vi "Add Cell.vi"(8 "error in":errorcluster, 10 "Cell Address":string, 11 "Row in":refnum<k24>) -> (0 "error out":errorcluster, 2 "Cell":refnum<k24>, 3 "Row out":refnum<k24>)   [LabVIEW 2019, in "Open Xml.lvlib"]
uses:
  Open Xml.lvlib
  D:/git/Open-Xml-LabVIEW/Source/DocumentFormat.OpenXml.dll
  DocumentFormat.OpenXml.dll
  D:/git/Open-Xml-LabVIEW/Source/DocumentFormat.OpenXml.Framework.dll
  DocumentFormat.OpenXml.Framework.dll
  D:/git/Open-Xml-LabVIEW/Source/OpenXmlGenericsWrapper.dll
  OpenXmlGenericsWrapper.dll
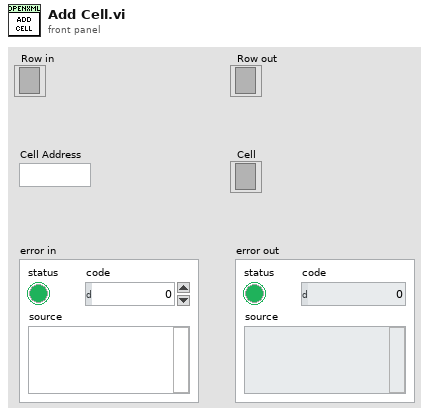
[diagram p1: front panel]
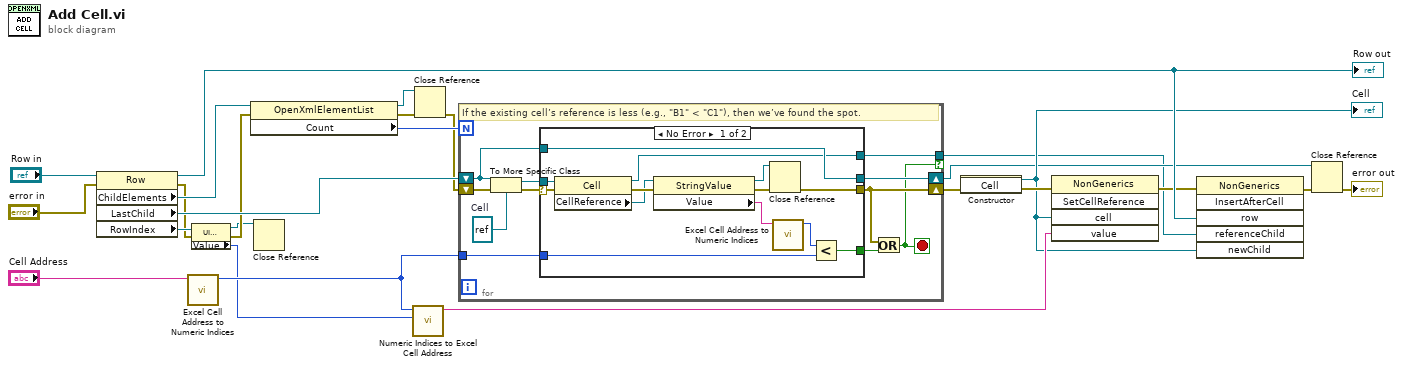
[diagram p0: block diagram]
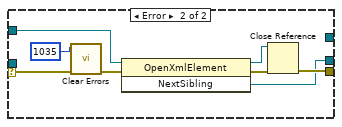
[diagram p2: hidden frame]
diagram:
  n1 = property class="Row"(reference="Row in", error in="error in") -> (reference out=w16:refnum<k24>, error out=w9:errorcluster, "ChildElements"=w24:refnum<k24>, "LastChild"=w22:refnum<k24>, "RowIndex"=w10:refnum<k24>)
  "Row out" <- w16
  n2 = call "Excel Cell Address to Numeric Indices.vi"("Cell Name"="Cell Address") -> ("Column Number"=w11:i32)  [unwired: 9 in, 1 out]
  n3 = property class="UInt32Value"(reference=w10, error in=w9) -> (reference out=w5:refnum<k24>, error out=w8:errorcluster, "Value"=w7:u32)
  n4 = property class="OpenXmlElementList"(reference=w24, error in=w8) -> (reference out=w17:refnum<k24>, error out=w21:errorcluster, "Count"=w23:i32)
  n5 = Close Reference(reference=w5) -> ()  [unwired: 1 in, 1 out]
  n6 = call "Numeric Indices to Excel Cell Address.vi"("Row"=w7, "Column"=w11) -> ("Cell Address"=w6:string)  [unwired: 9 in]
  n7 = Close Reference(reference=w17, error in (no error)=w21) -> (error out=w18:errorcluster)
  n8 = for {
    N: w23 -> [_]
    tunnel: w11 -> [w30]
    shift-right: [w29] -> w3
    shift-left: w22 -> [w31]
    tunnel: [w28] -> w2 if=w27
    shift-right: [w33] -> w13
    shift-left: w18 -> [w34]
    stop <- w27 stop-if-true
    w35 = refnum<k24> refnum  # Cell
    # "If the existing cell’s reference is less (e.g., \"B1\" < \"C1\"), then we’ve found the spot."
    n9 = To More Specific Class(target class=w35, reference=w31, error in=w34) -> (specific class reference=w32:refnum<k24>, error out=w36:errorcluster)
    n10 = case shown="No Error" w36 {
      selector: w36 -> [w49 w57]
      tunnel: [w38 w51] -> w33
      tunnel: w32 -> [w48 _]
      tunnel: w31 -> [w40 w54]
      tunnel: w30 -> [w44 _]
      tunnel: [w41 _] -> w26
      tunnel: [w40 w50] -> w29
      tunnel: [w39 _] -> w28
      frame No Error {
        n11 = property class="Cell"(reference=w48, error in=w49) -> (reference out=w39:refnum<k24>, error out=w47:errorcluster, "CellReference"=w46:refnum<k24>)
        n12 = property class="StringValue"(reference=w46, error in=w47) -> (reference out=w37:refnum<k24>, error out=w43:errorcluster, "Value"=w45:string)
        n13 = Close Reference(reference=w37, error in (no error)=w43) -> (error out=w38:errorcluster)
        n14 = call "Excel Cell Address to Numeric Indices.vi"("Cell Name"=w45) -> ("Column Number"=w42:i32)  [unwired: 9 in, 1 out]
        n15 = Less?(x=w42, y=w44) -> (x < y?=w41:bool)
      }
      frame Error {
        n16 = call <vilib>:"Clear Errors.vi"("error in (no error)"=w57, "specific error code to clear (0: all)"=1035) -> ("error out"=w55:errorcluster)  [unwired: 4 in, 1 out]
        n17 = invoke class="OpenXmlElement" method="NextSibling"(reference=w54, error in=w55) -> (reference out=w53:refnum<k24>, error out=w52:errorcluster, "NextSibling"=w50:refnum<k24>)  [unwired: 1 in]
        n18 = Close Reference(reference=w53, error in (no error)=w52) -> (error out=w51:errorcluster)
      }
    }
    n19 = Or(x=w33, y=w26) -> (x .or. y?=w27:bool)
  }
  n20 = constructor class="Cell"(error in=w13) -> (reference out=w4:refnum<k24>, error out=w20:errorcluster)  [unwired: 2 in, 1 out]
  "Cell" <- w4
  n21 = invoke class="NonGenerics" method="SetCellReference"(error in=w20, "cell"=w4, "value"=w6) -> (error out=w12:errorcluster)  [unwired: 2 in, 4 out]
  n22 = invoke class="NonGenerics" method="InsertAfterCell"(error in=w12, "row"=w16, "referenceChild"=w2, "newChild"=w4) -> (error out=w14:errorcluster)  [unwired: 2 in, 5 out]
  n23 = Close Reference(reference=w3, error in (no error)=w14) -> (error out=→"error out":errorcluster)
